vi "CM-TDT-Endpoint To Sequential Connection Number (1D String).vi"(0 "Path In":path, 5 "Endpoints":string[](array[string]), 9 "Section":string, 11 "error in (no error)":errorcluster, 12 "Front panel only":bool) -> (4 "Path Out":path, 8 "SeqCxnNum":i32[](array[numeric]), 15 "error out":errorcluster)   [LabVIEW 2020]
uses:
  PXI DAQ VIs/TDT VIs/Typedefs/TDT-Input source.ctl
  <vilib>/Utility/config.llb/Read Key (String).vi
  <vilib>/Utility/config.llb/NI_LVConfig.lvlib
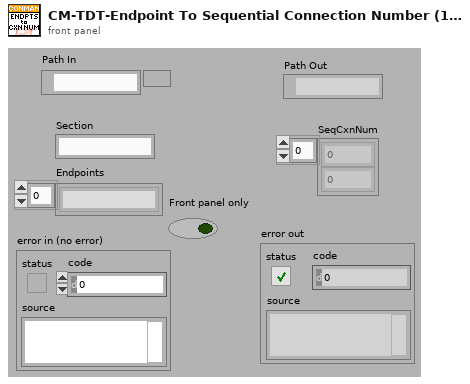
[diagram p1: front panel]
types:
  T1 = typedef "TDT-Input source.ctl" = enum16{"Front Panel", "RA4LI", "RA16LI"}
  T2 = typedef "TDT-Device Config.ctl" = cluster{"Output":T3, "Input":T1}
  T3 = typedef "TDT-Output source.ctl" = cluster{"Device":T4, "Num":i32}
  T4 = typedef "TDT-Device ID.ctl" = enum16{"None", "PA5", "RP2", "RL2", "RA16", "RV8", "RX5", "RX6", "RX7", "RX8", "RZ2", "RZ5", "RZ6"}
  T5 = typedef "NI_LVConfig.lvlib/Config Data RefNum.ctl" = refnum<k1>
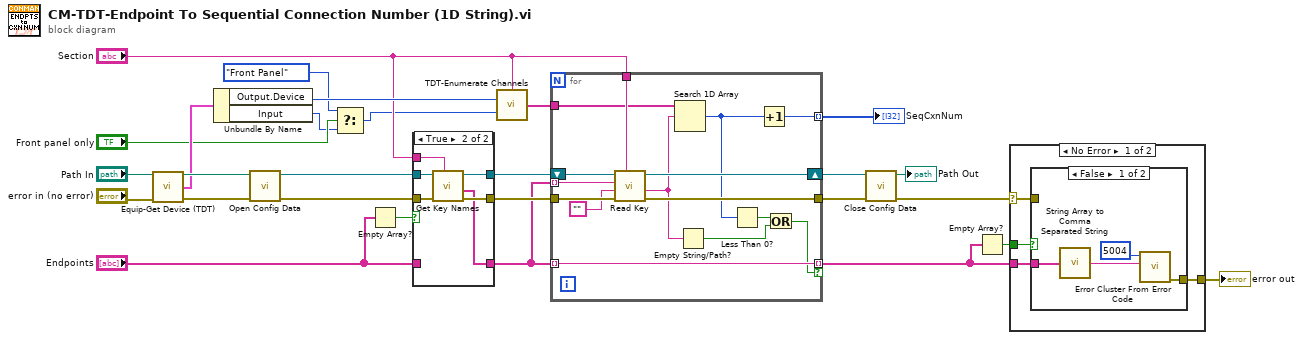
[diagram p0: block diagram]
diagram:
  n1 = call "Equip-Get Device (TDT).vi"("Path In"="Path In", "error in (no error)"="error in (no error)") -> ("Path Out"=w19:path, "TDT-Device Config"=w16:T2, "error out"=w18:errorcluster)  [unwired: 11 in]
  n2 = Unbundle By Name(w16) -> ("Output.Device"=w24:T4, "Input"=w4:T1)
  n3 = call <vilib>:"Open Config Data.vi"("error in (no error)"=w18, "configuration file path"=w19) -> ("error out"=w14:errorcluster, "refnum"=w15:T5)  [unwired: 7 in, 1 out]
  n4 = Select(t=TDT-Input_source."Front Panel", s="Front panel only", f=w4) -> (s? t:f=w2:T1)
  n5 = Empty Array?(array="Endpoints") -> (empty?=w10:bool)
  n6 = case shown="True" w10 {
    tunnel: w14 -> [w29 w36]
    tunnel: w15 -> [w30 w35]
    tunnel: [w30 w34] -> w13
    tunnel: [w29 w33] -> w12
    tunnel: "Section" -> [_ w32]
    tunnel: "Endpoints" -> [w28 _]
    tunnel: [w28 w31] -> w8
    frame False {
    }
    frame True {
      n7 = call <vilib>:"Get Key Names.vi"("section"=w32, "error in (no error)"=w36, "refnum"=w35) -> ("error out"=w33:errorcluster, "key names"=w31:string[], "refnum out"=w34:T5)  [unwired: 5 in, 1 out]
    }
  }
  n8 = call "TDT-Enumerate Channels.vi"("Type"="Section", "IO Device"=w24, "Input"=w2) -> ("IO Channels"=w23:string[])  [unwired: 12 in]
  n9 = for {
    tunnel: w12 -> [w49]
    tunnel: w8 -> [w50] mode=indexing
    tunnel: "Section" -> [w47]
    tunnel: [w45] -> w25
    shift-right: [w46] -> w26
    shift-left: w13 -> [w51]
    tunnel: w23 -> [w44]
    tunnel: [w37] -> w22 mode=indexing
    tunnel: [w43] -> w7 mode=indexing if=w38
    tunnel: w8 -> [w43] mode=indexing
    n10 = call-poly <vilib>:"Read Key.vi"("section"=w47, "error in (no error)"=w49, "default value"="", "key"=w50, "refnum"=w51) -> ("error out"=w45:errorcluster, "value"=w42:string, "refnum out"=w46:T5)  [unwired: 3 in, 1 out]
    n11 = Search 1D Array(1D array=w44, element=w42) -> (index of element=w41:i32)  [unwired: 1 in]
    n12 = Empty String/Path?(string/path=w42) -> (empty?=w39:bool)
    n13 = Less Than 0?(x=w41) -> (x < 0?=w40:bool)
    n14 = Increment(x=w41) -> (x+1=w37:i32)
    n15 = Or(x=w40, y=w39) -> (x .or. y?=w38:bool)
  }
  "SeqCxnNum" <- w22
  n16 = call <vilib>:"Close Config Data.vi"("error in (no error)"=w25, "refnum"=w26) -> ("error out"=w21:errorcluster, "file path"=→"Path Out":path)  [unwired: 8 in]
  n17 = Empty Array?(array=w7) -> (empty?=w6:bool)
  n18 = case shown="No Error" w21 {
    selector: w21 -> [w54 w61]
    tunnel: [w55 w61] -> w20
    tunnel: w7 -> [w53 _]
    tunnel: w6 -> [w52 _]
    frame No Error {
      n19 = case shown="False" w52 {
        tunnel: w54 -> [_ w60]
        tunnel: [w59 w60] -> w55
        tunnel: w53 -> [w57 _]
        frame False {
          n20 = call "String Array to Comma Separated String.vi"("String Array"=w57) -> ("comma separated string"=w56:string)
          n21 = call <vilib>:"Error Cluster From Error Code.vi"("error message (\"\")"=w56, "error code (0)"=5004) -> ("error out"=w59:errorcluster)  [unwired: 7 in]
        }
        frame True {
        }
      }
    }
    frame Error {
    }
  }
  "error out" <- w20
